vi "Generate_SubVI_from_path.vi"(8 "error in (no error)":errorcluster, 9 "location":T1, 10 "path":path, 11 "VI in":refnum<vi>) -> (0 "error out":errorcluster, 3 "SubVI out":refnum<vi>)   [LabVIEW 2025]
uses:
  <vilib>/Utility/miscctls.llb/LVPointTypeDef.ctl
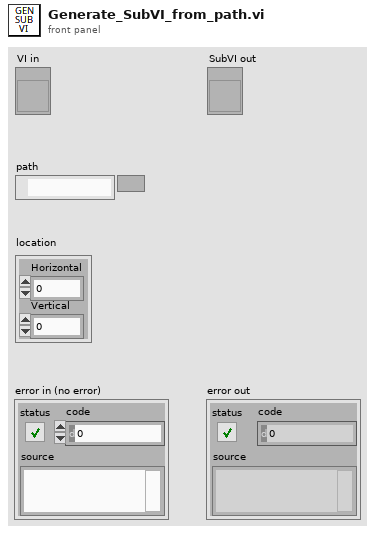
[diagram p1: front panel]
types:
  T1 = typedef "LVPointTypeDef.ctl" = cluster{"Horizontal":i16, "Vertical":i16}
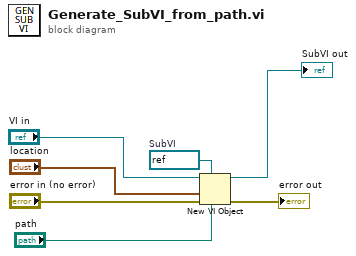
[diagram p0: block diagram]
diagram:
  w1 = refnum<vi> refnum  # SubVI
  n1 = New VI Object(vi object class=w1, owner refnum="VI in", position/next to="location", 6:"path", 8:"error in (no error)") -> (object refnum=→"SubVI out":refnum<vi>, 0:→"error out":errorcluster)  [unwired: 3 in]
